vi "Configure Local Remote.vi"(7 "Slave Address":i32=-1 min=-1 max=30 step=1, 8 "error":errorcluster, 10 "Mode":enum16{"LOCAL", "REMOTE", "LOCKOUT"}(ring), 11 "VISA":refnum<visa-resource-name>) -> (0 "error out":errorcluster, 3 "VISA out":refnum<visa-resource-name>)   [LabVIEW 2025, in "TDK-Lambda GEN LAN Series.lvlib"]
doc: "Configure the operating mode of the power supply to front-panel or remote (LAN). The input enumerated type may be:\n\n(0) Local (Default). The power-supply settings are made from its front panel buttons and knobs \n(1) Remote. The power-supply settings are made using the LAN port. The front panel may be used to view settings but not change them. The \"REM/LOC\" button may be pressed to set local mode\n(2) Local Lockout. Same as Remote but the \"REM/LOC\" button will not operate\n\nNote: when in Local mode, any LAN command that changes the instrument's output state will put the instrument into remote"
uses:
  <userlib>/TDK-Lambda GEN LAN Series/TDK-Lambda GEN LAN Series.lvlib
panel:
  # "TDK-Lambda Genesys \n LAN\n  DC Power Supplies"
  # "Set Modes:\n Local, Remote, or Lockout"
  # "(c) 2019 TDK-Lambda.  ALL RIGHTS RESERVED."
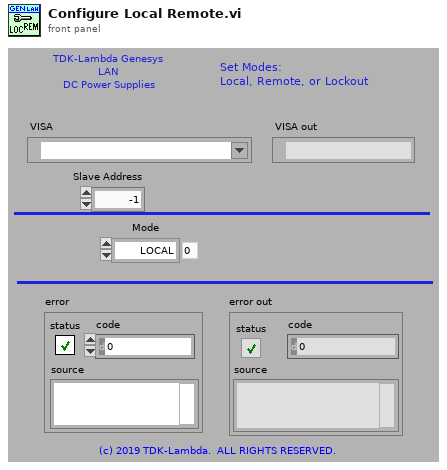
[diagram p1: front panel]
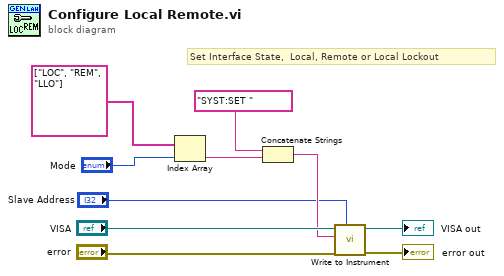
[diagram p0: block diagram]
diagram:
  # "Set Interface State,  Local, Remote or Local Lockout"
  n1 = Index Array(array=string[] ["LOC", "REM", "LLO"], index="Mode") -> (element=w4:string)
  n2 = Concatenate Strings("SYST:SET ", w4) -> (w2:string)
  n3 = call <userlib>:"Write to Instrument.vi"("Slave Address"="Slave Address", "error"="error", "Command"=w2, "VISA"="VISA") -> ("error out"=→"error out":errorcluster, "VISA out"=→"VISA out":refnum<visa-resource-name>)  [unwired: 6 in]
